vi "Wait Start.vi"(5 "Sequence Control":T1, 8 "error in (no error)":errorcluster, 11 "State in":refnum<class "State.lvclass">) -> (0 "error out":errorcluster, 1 "Close":bool, 2 "Start":bool, 3 "State out":refnum<class "State.lvclass">)   [LabVIEW 2020, in "VolatusSeq.lvlib" / "State.lvclass"]
uses:
  State.lvclass
  State.lvclass/State.ctl
  Sequence Time.ctl
  VolatusSeq.lvlib
  State Control.ctl
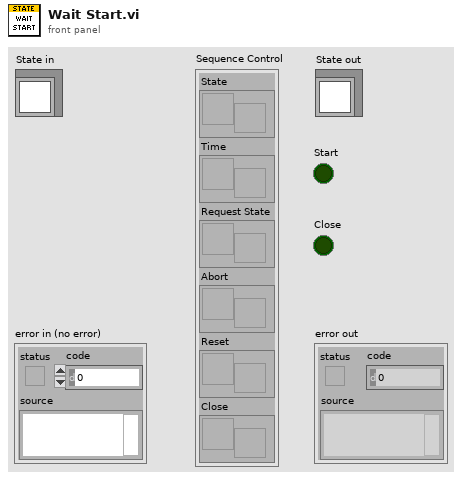
[diagram p1: front panel]
types:
  T1 = typedef "VolatusSeq.lvlib/State Control.ctl" = cluster{"State":refnum<notifier>, "Time":refnum<notifier>, "Request State":refnum<notifier>, "Abort":refnum<notifier>, "Reset":refnum<notifier>, "Close":refnum<notifier>}
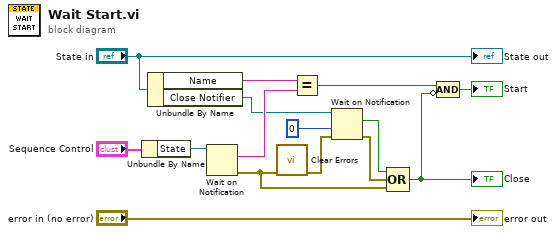
[diagram p0: block diagram]
diagram:
  n1 = Unbundle By Name("Sequence Control") -> ("State"=w13:refnum<notifier>)
  n2 = Unbundle By Name("State in") -> ("Name"=w11:string, "Close Notifier"=w7:refnum<notifier>)
  n3 = Wait on Notification(notifier=w13) -> (notification=w10:string, error out=w5:errorcluster)  [unwired: 3 in, 2 out]
  n4 = call <vilib>:"Clear Errors.vi"("error in (no error)"=w5) -> ("error out"=w8:errorcluster)  [unwired: 5 in, 1 out]
  n5 = Equal?(x=w11, y=w10) -> (x = y?=w9:bool)
  n6 = Wait on Notification(notifier=w7, timeout in ms (-1)=0, error in (no error)=w8) -> (notification=w3:bool, error out=w4:errorcluster)  [unwired: 1 in, 2 out]
  n7 = Compound Arithmetic op=OR(w3, w4, w5) -> (w1:bool)
  "Close" <- w1
  n8 = Compound Arithmetic op=AND(w9, invert w1) -> (→"Start":bool)
  "error out" <- "error in (no error)"
  "State out" <- "State in"
